vi "multi_pos.vi"() -> ()   [LabVIEW 2023]
uses:
  <vilib>/Python/Open Venv Python Session.vi
  <instrlib>/Phidgets/Phidget Voltage Ratio Input/Phidget Voltage Ratio Input.lvlib
  <instrlib>/Phidgets/Phidget Common/Phidget Common.lvlib
  <instrlib>/Phidgets/Phidget Voltage Ratio Input/Public/VoltageRatioInputClose.vi
  <instrlib>/Phidgets/Phidget Voltage Ratio Input/Public/VoltageRatioInputStart.vi
panel:
  in  "IsHubPort 2":bool caption="IsHubPort"
  out "Serial Number Return 2":i32 caption="Serial Number Return"
  in  "Device Info 2":T1={"Serial Number"=-1, "Channel"=0, "Port"=0} caption="Device Info"
  out "error out 2":errorcluster caption="error out"
  in  "stop 4":bool caption="stop"
  out "Voltage Ratio 2":dbl caption="Voltage Ratio" format="%_4g"
  out "Close session error 2":errorcluster
  out "start error 2":errorcluster
  out "iter 2":dbl
  in  "stop 3":bool
  in  "torque input 2":dbl
  out "torque 2":dbl
  in  "Move pos input 2":dbl
  in  "Enum 3":enum16{"hold", "get_pos", "move", "torque"}(ring)
  out "pos 2":dbl
  out "main error  2":errorcluster
  in  "IsHubPort":bool
  out "Serial Number Return":i32
  in  "Device Info":T1={"Serial Number"=-1, "Channel"=0, "Port"=0}
  out "error out":errorcluster
  in  "stop 2":bool caption="stop"
  out "Voltage Ratio":dbl format="%_4g"
  out "Close session error":errorcluster
  out "start error":errorcluster
  out "iter":dbl
  in  "stop":bool
  in  "torque input":dbl
  out "torque":dbl
  in  "Move pos input":dbl
  in  "Enum 2":enum16{"hold", "get_pos", "move", "torque"}(ring)
  out "pos":dbl
  out "main error":errorcluster
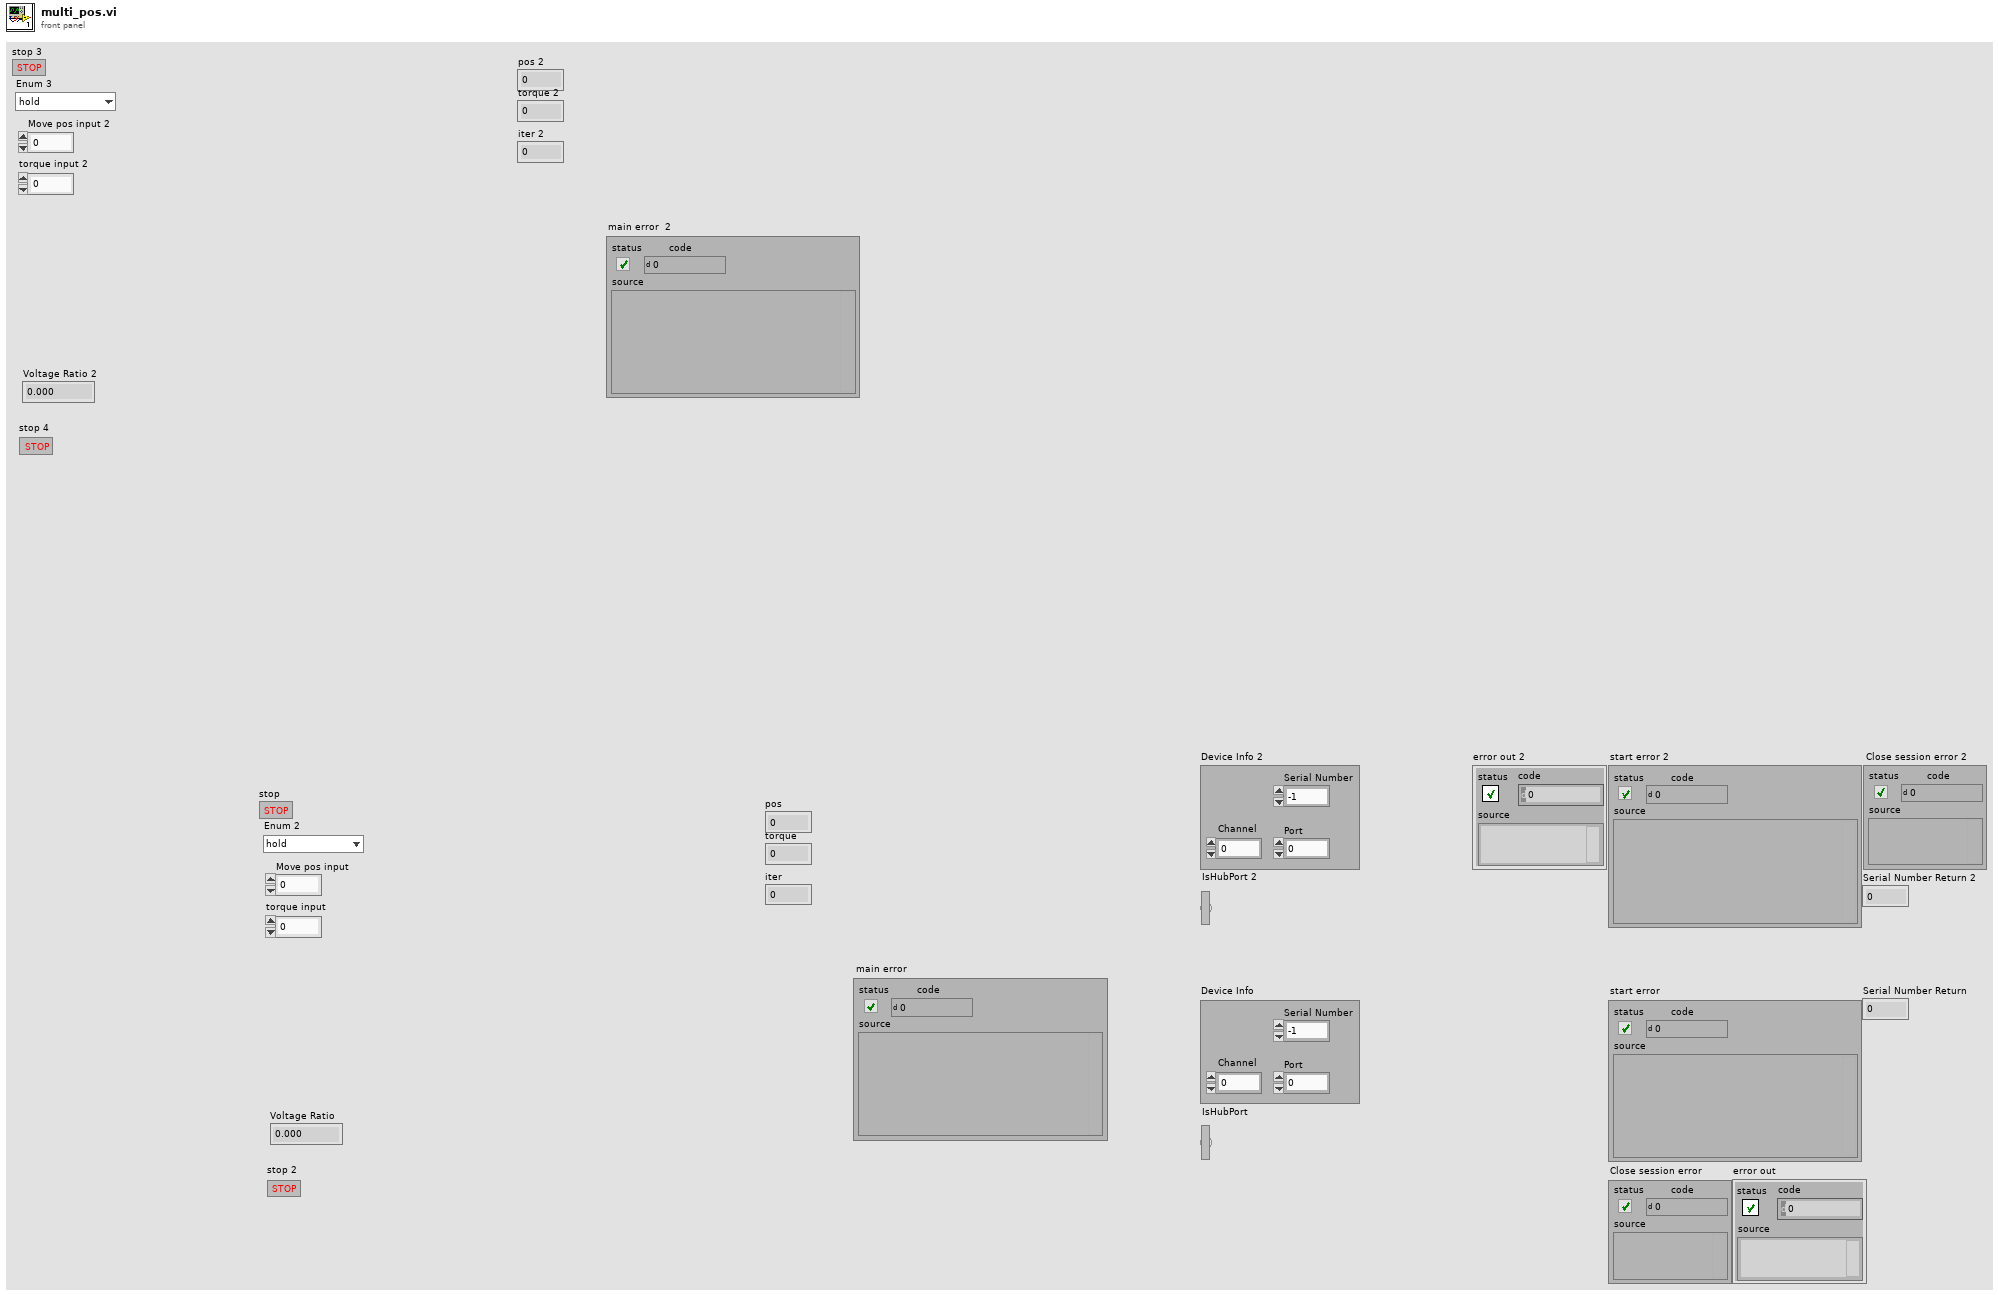
[diagram p1: front panel]
types:
  T1 = cluster{"Serial Number":i32, "Channel":i32, "Port":i32}
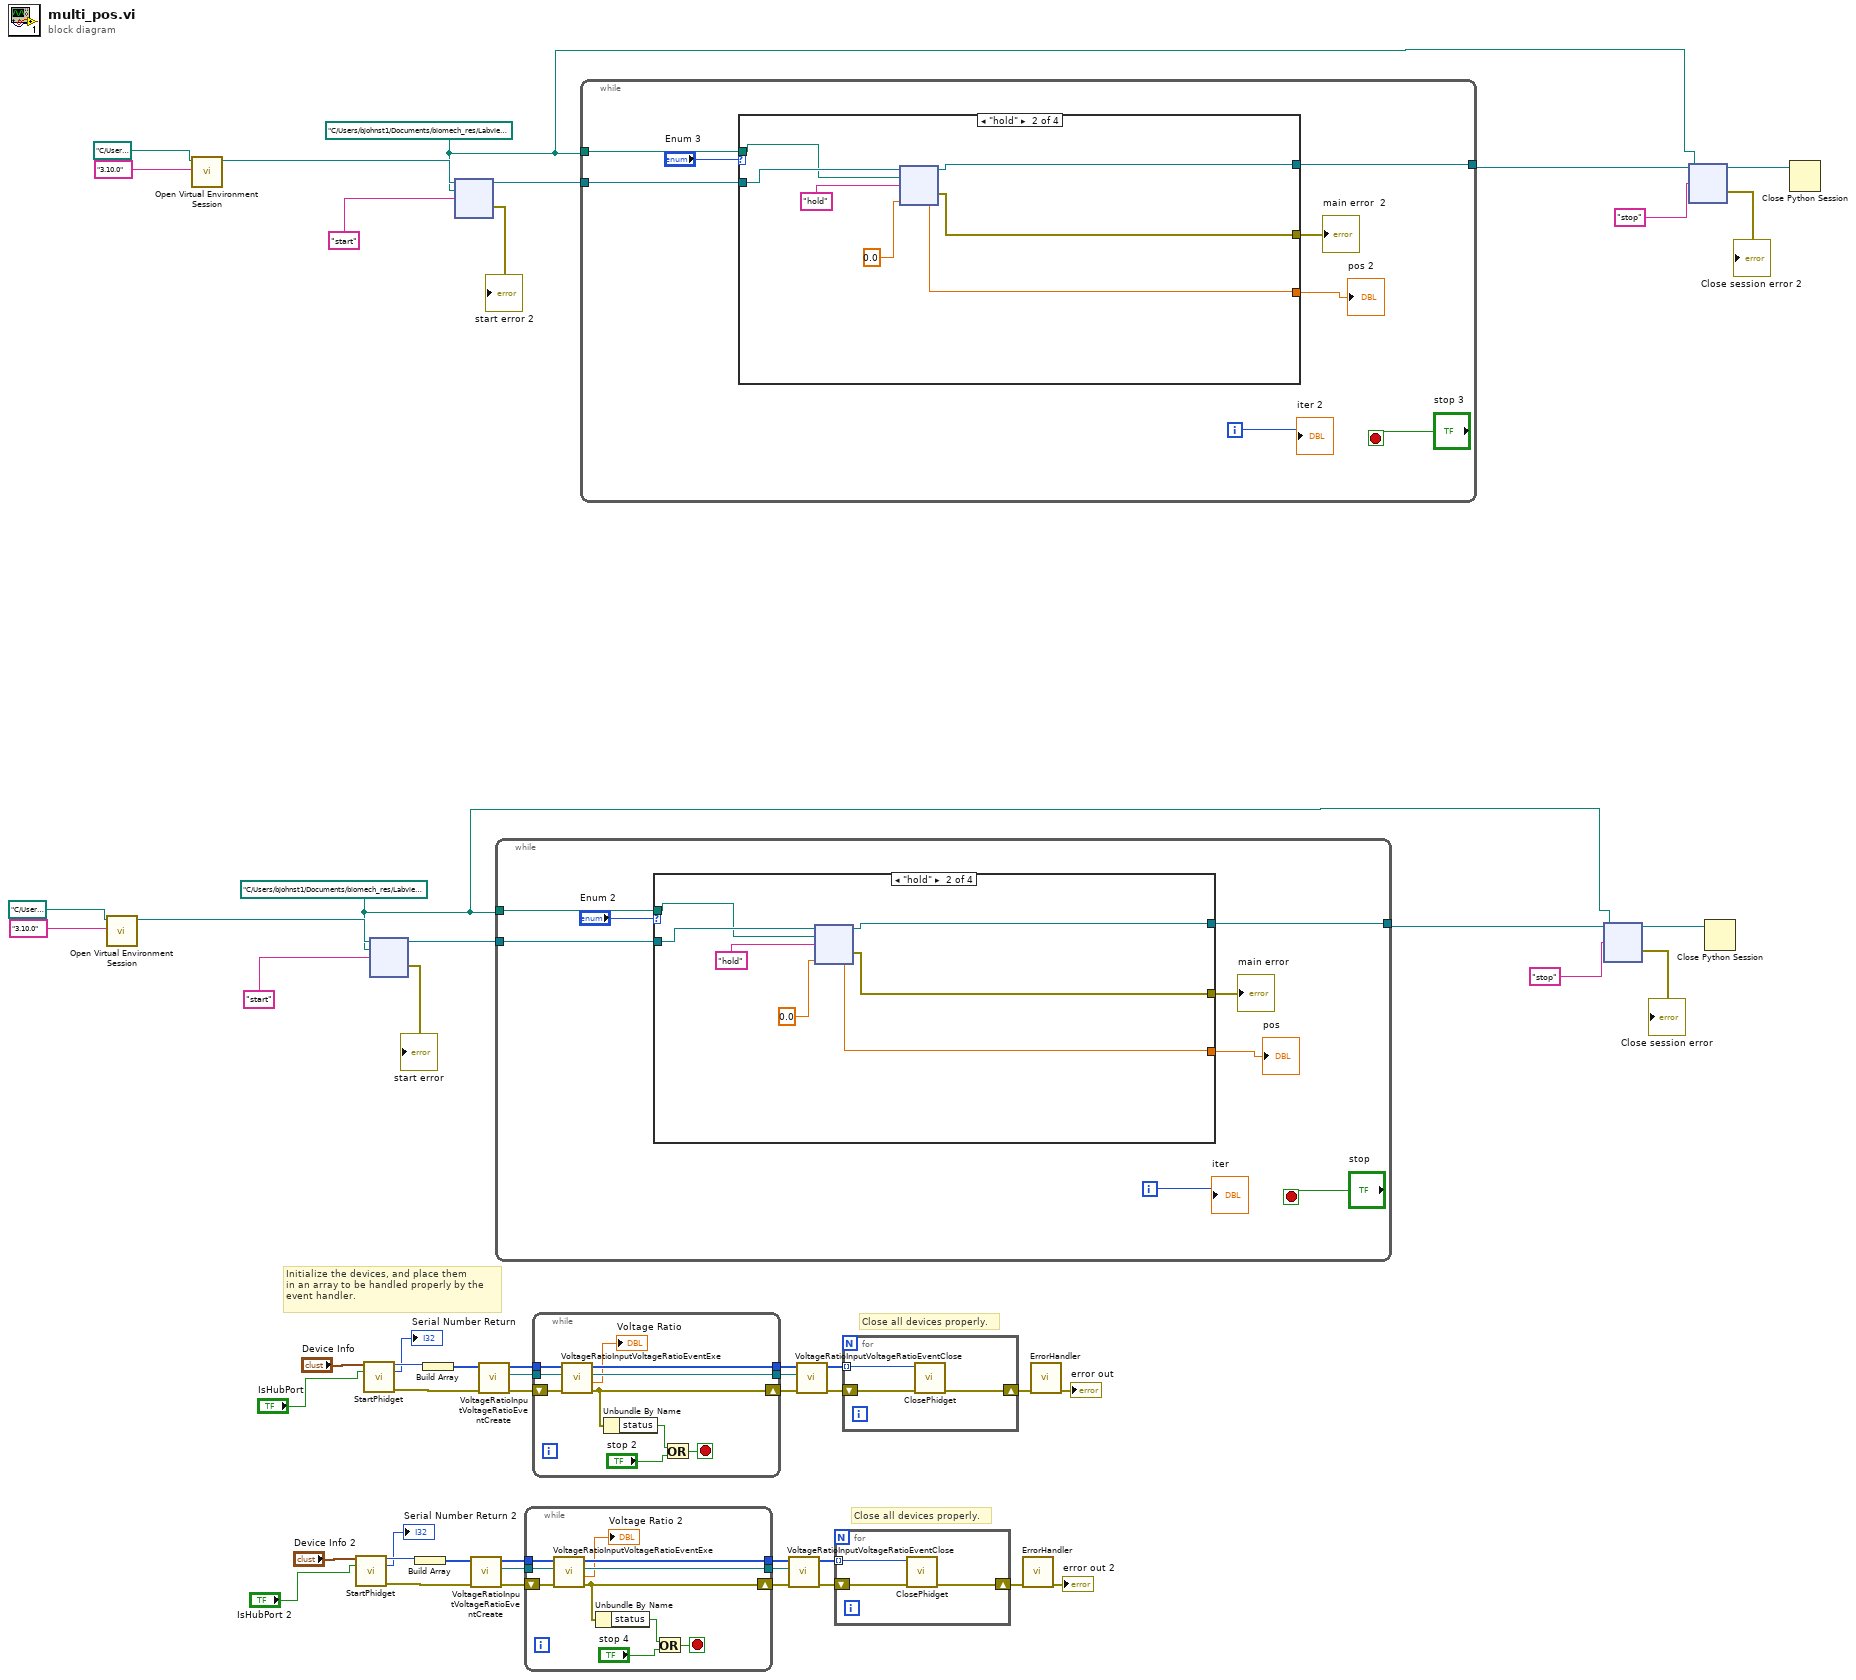
[diagram p0: block diagram]
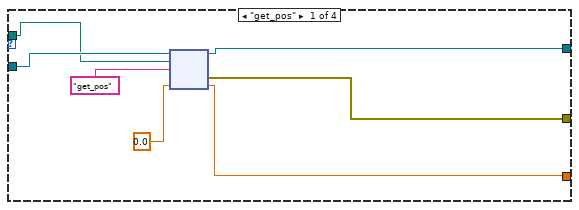
[diagram p2: hidden frame]
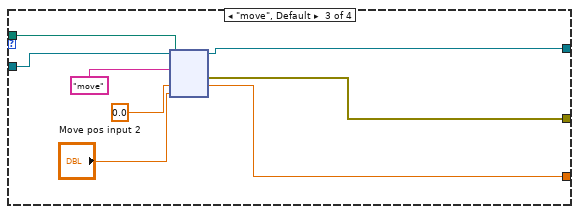
[diagram p3: hidden frame]
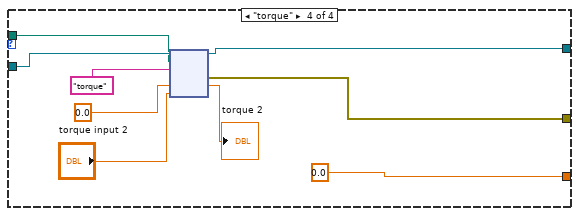
[diagram p4: hidden frame]
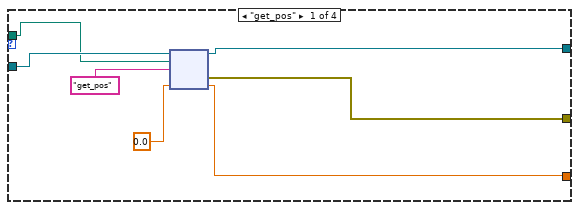
[diagram p5: hidden frame]
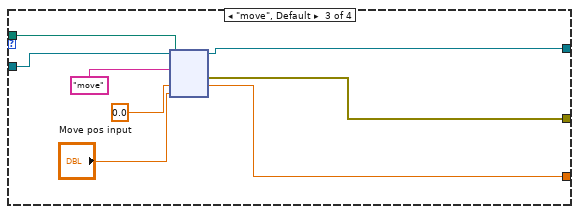
[diagram p6: hidden frame]
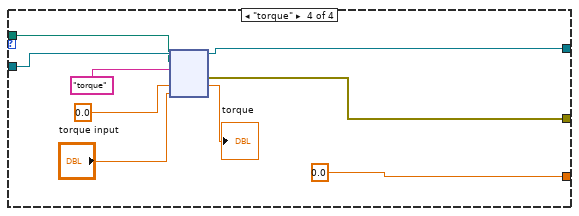
[diagram p7: hidden frame]
diagram:
  w17 = path "C:/Users/bjohnst1/Documents/biomech_res/Labview/labview_moteus_funcs.py"
  w44 = path "C:/Users/bjohnst1/Documents/biomech_res/Labview/labview_moteus_funcs.py"
  # "Close all devices properly."
  # "Close all devices properly."
  # "Initialize the devices, and place them\nin an array to be handled properly by the\nevent handler."
  n1 = call-poly <vilib>:"Open Virtual Environment Session.vi"("Python version"="3.10.0", "Env path"=path "C:/Users/bjohnst1/Documents/biomech_res/res_env2") -> ("session out"=w50:refnum<k35>)  [unwired: 8 in, 1 out]
  n2 = call-poly <vilib>:"Open Virtual Environment Session.vi"("Python version"="3.10.0", "Env path"=path "C:/Users/bjohnst1/Documents/biomech_res/res_env2") -> ("session out"=w23:refnum<k35>)  [unwired: 8 in, 1 out]
  n3 = call-poly <instrlib>:"StartPhidget.vi"("Device Info"="Device Info 2", "IsHubPort"="IsHubPort 2") -> ("Phidget ID"=w6:u64, "Serial Number Return"=→"Serial Number Return 2":i32, "error out"=w2:errorcluster)  [unwired: 10 in, 1 out]
  n4 = call-poly <instrlib>:"StartPhidget.vi"("Device Info"="Device Info", "IsHubPort"="IsHubPort") -> ("Phidget ID"=w33:u64, "Serial Number Return"=→"Serial Number Return":i32, "error out"=w29:errorcluster)  [unwired: 10 in, 1 out]
  n5 = node(w50, w44, "start") -> (w49:refnum<k35>, →"start error":errorcluster)  [unwired: 3 in, 2 out]
  n6 = Build Array(w6) -> (w16:u64[])
  n7 = Build Array(w33) -> (w43:u64[])
  n8 = node(w23, w17, "start") -> (w22:refnum<k35>, →"start error 2":errorcluster)  [unwired: 3 in, 2 out]
  n9 = call <instrlib>:"VoltageRatioInputVoltageRatioEventCreate.vi"("error in (no error)"=w2, "Devices In"=w16) -> ("error out"=w9:errorcluster, "Event Registration Refnum"=w14:refnum<event-registration>, "Devices Out"=w15:u64[])  [unwired: 7 in]
  n10 = call <instrlib>:"VoltageRatioInputVoltageRatioEventCreate.vi"("error in (no error)"=w29, "Devices In"=w43) -> ("error out"=w36:errorcluster, "Event Registration Refnum"=w41:refnum<event-registration>, "Devices Out"=w42:u64[])  [unwired: 7 in]
  n11 = while {
    tunnel: [w61] -> w48
    tunnel: w49 -> [w59]
    tunnel: w44 -> [w58]
    i -> [w62]
    stop <- "stop" stop-if-true
    n12 = case shown="\"hold\"" "Enum 2" {
      tunnel: [w69 w76 w84 w93] -> w61
      tunnel: w59 -> [w67 w74 w82 w91]
      tunnel: [w65 w72 w79 0.0] -> w56
      tunnel: [w64 w71 w78 w89] -> w55
      tunnel: w58 -> [w63 w70 w77 w85]
      frame "get_pos" {
        n13 = node(w67, w63, "get_pos", 0.0) -> (w69:refnum<k35>, w64:errorcluster, w65:dbl)  [unwired: 1 in, 2 out]
      }
      frame "hold" {
        n14 = node(w74, w70, "hold", 0.0) -> (w76:refnum<k35>, w71:errorcluster, w72:dbl)  [unwired: 1 in, 2 out]
      }
      frame "move", Default {
        n15 = node(w82, w77, "move", 0.0, "Move pos input") -> (w84:refnum<k35>, w78:errorcluster, w79:dbl)  [unwired: 2 in, 2 out]
      }
      frame "torque" {
        n16 = node(w91, w85, "torque", 0.0, "torque input") -> (w93:refnum<k35>, w89:errorcluster, →"torque":dbl)  [unwired: 2 in, 2 out]
      }
    }
    "pos" <- w56
    "main error" <- w55
    "iter" <- w62
  }
  n17 = while {
    tunnel: w15 -> [w103]
    tunnel: w14 -> [w99]
    tunnel: [w102] -> w11
    shift-right: [w98] -> w10
    shift-left: w9 -> [w101]
    tunnel: [w100] -> w4
    stop <- w97 stop-if-true
    n18 = call <instrlib>:"VoltageRatioInputVoltageRatioEventExe.vi"("error in (no error)"=w101, "Event Registration Refnum In"=w99, "Devices In"=w103) -> ("error out"=w98:errorcluster, "VoltageRatio"=→"Voltage Ratio 2":dbl, "Event Registration Refnum Out"=w102:refnum<event-registration>, "Devices Out"=w100:u64[])  [unwired: 2 in, 3 out]
    n19 = Unbundle By Name(w98) -> ("status"=w95:bool)
    n20 = Or(x=w95, y="stop 4") -> (x .or. y?=w97:bool)
  }
  n21 = while {
    tunnel: w42 -> [w113]
    tunnel: w41 -> [w109]
    tunnel: [w112] -> w38
    shift-right: [w108] -> w37
    shift-left: w36 -> [w111]
    tunnel: [w110] -> w31
    stop <- w107 stop-if-true
    n22 = call <instrlib>:"VoltageRatioInputVoltageRatioEventExe.vi"("error in (no error)"=w111, "Event Registration Refnum In"=w109, "Devices In"=w113) -> ("error out"=w108:errorcluster, "VoltageRatio"=→"Voltage Ratio":dbl, "Event Registration Refnum Out"=w112:refnum<event-registration>, "Devices Out"=w110:u64[])  [unwired: 2 in, 3 out]
    n23 = Unbundle By Name(w108) -> ("status"=w105:bool)
    n24 = Or(x=w105, y="stop 2") -> (x .or. y?=w107:bool)
  }
  n25 = while {
    tunnel: [w120] -> w21
    tunnel: w22 -> [w118]
    tunnel: w17 -> [w117]
    i -> [w121]
    stop <- "stop 3" stop-if-true
    n26 = case shown="\"hold\"" "Enum 3" {
      tunnel: [w128 w135 w143 w152] -> w120
      tunnel: w118 -> [w126 w133 w141 w150]
      tunnel: [w124 w131 w138 0.0] -> w115
      tunnel: [w123 w130 w137 w148] -> w114
      tunnel: w117 -> [w122 w129 w136 w144]
      frame "get_pos" {
        n27 = node(w126, w122, "get_pos", 0.0) -> (w128:refnum<k35>, w123:errorcluster, w124:dbl)  [unwired: 1 in, 2 out]
      }
      frame "hold" {
        n28 = node(w133, w129, "hold", 0.0) -> (w135:refnum<k35>, w130:errorcluster, w131:dbl)  [unwired: 1 in, 2 out]
      }
      frame "move", Default {
        n29 = node(w141, w136, "move", 0.0, "Move pos input 2") -> (w143:refnum<k35>, w137:errorcluster, w138:dbl)  [unwired: 2 in, 2 out]
      }
      frame "torque" {
        n30 = node(w150, w144, "torque", 0.0, "torque input 2") -> (w152:refnum<k35>, w148:errorcluster, →"torque 2":dbl)  [unwired: 2 in, 2 out]
      }
    }
    "pos 2" <- w115
    "main error  2" <- w114
    "iter 2" <- w121
  }
  n31 = call <instrlib>:"VoltageRatioInputVoltageRatioEventClose.vi"("error in (no error)"=w10, "Event Registration Refnum In"=w11, "Devices In"=w4) -> ("error out"=w7:errorcluster, "Devices Out"=w5:u64[])  [unwired: 7 in]
  n32 = call <instrlib>:"VoltageRatioInputVoltageRatioEventClose.vi"("error in (no error)"=w37, "Event Registration Refnum In"=w38, "Devices In"=w31) -> ("error out"=w34:errorcluster, "Devices Out"=w32:u64[])  [unwired: 7 in]
  n33 = for {
    tunnel: w5 -> [w153] mode=indexing
    shift-right: [w155] -> w13
    shift-left: w7 -> [w154]
    n34 = call-poly <instrlib>:"ClosePhidget.vi"("error in"=w154, "Device In"=w153) -> ("error out"=w155:errorcluster)  [unwired: 9 in]
  }
  n35 = for {
    tunnel: w32 -> [w156] mode=indexing
    shift-right: [w158] -> w40
    shift-left: w34 -> [w157]
    n36 = call-poly <instrlib>:"ClosePhidget.vi"("error in"=w157, "Device In"=w156) -> ("error out"=w158:errorcluster)  [unwired: 9 in]
  }
  n37 = call <instrlib>:"ErrorHandler.vi"("error in"=w13) -> ("error out"=→"error out 2":errorcluster)  [unwired: 9 in, 1 out]
  n38 = call <instrlib>:"ErrorHandler.vi"("error in"=w40) -> ("error out"=→"error out":errorcluster)  [unwired: 9 in, 1 out]
  n39 = node(w48, w44, "stop") -> (w47:refnum<k35>, →"Close session error":errorcluster)  [unwired: 3 in, 2 out]
  n40 = node(w21, w17, "stop") -> (w20:refnum<k35>, →"Close session error 2":errorcluster)  [unwired: 3 in, 2 out]
  n41 = Close Python Session(session in=w47) -> ()  [unwired: 1 in, 1 out]
  n42 = Close Python Session(session in=w20) -> ()  [unwired: 1 in, 1 out]
